vi "Subtask1_Marble_Project.vi"() -> ()   [LabVIEW 2016]
uses:
  <vilib>/NXT/Block Support/NXT_InputPort.ctl
  <vilib>/NXT/Block Support/NXT_OutputPort.ctl
  <vilib>/NXT/Dual Mode Library/Sensors/Touch_Pressed.vi
  <vilib>/NXT/Dual Mode Library/Sensors/Touch_Bumped.vi
  <vilib>/NXT/NXTIO Xnodes/NXTIONodeSubVIs/NXTMoveMotors.vi
  <vilib>/NXT/NXTIO Xnodes/AddressXNode/NXTIOAddress.xnode
  <vilib>/NXT/NXTIO Xnodes/NXTIOXNode/NXTIO.xnode
  <vilib>/NXT/Subs/LVHSConnector.ctl
  <vilib>/NXT/LegoClasses/BrickReference/BrickReference.lvclass
panel:
  out "Motor Power":dbl
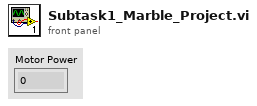
[diagram p1: front panel]
types:
  T1 = typedef "NXT_InputPort.ctl" = u32
  T2 = typedef "LVHSConnector.ctl" = refnum<class "BrickReference.lvclass">
  T3 = typedef "NXT_OutputPort.ctl" = u8
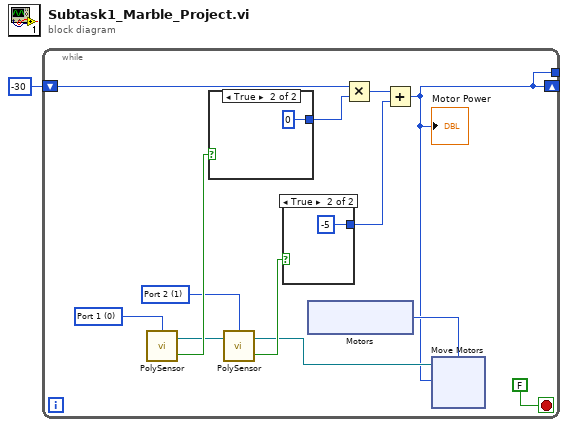
[diagram p0: block diagram]
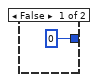
[diagram p2: hidden frame]
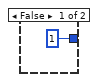
[diagram p3: hidden frame]
diagram:
  n1 = while {
    shift-right: [w2] -> _
    shift-left: -30 -> [w11]
    tunnel: [w2] -> _
    stop <- FALSE stop-if-true
    w6 = T1 1 items=["Port 1", "Port 2", "Port 3", "Port 4"] ("Port (Port 1)")
    w12 = T1 0 items=["Port 1", "Port 2", "Port 3", "Port 4"] ("Port (Port 1)")
    n2 = call-poly <vilib>:"PolySensor.vi"("Port (Port 1)"=w12) -> ("Yes / No"=w13:bool, "NXT/EV3"=w4:T2)  [unwired: 2 in]
    n3 = case shown="True" w13 {
      tunnel: [1 0] -> w10
      frame False {
      }
      frame True {
      }
    }
    n4 = call-poly <vilib>:"PolySensor.vi"("NXT/EV3"=w4, "Port (Port 1)"=w6) -> ("Yes / No"=w7:bool, "NXT/EV3"=w3:T2)  [unwired: 1 in]
    n5 = case shown="True" w7 {
      tunnel: [0 -5] -> w9
      frame False {
      }
      frame True {
      }
    }
    n6 = xnode "Motors"() -> ("Motor"=w14:T3)
    n7 = Multiply(x=w11, y=w10) -> (x*y=w8:i32)
    n8 = Add(x=w8, y=w9) -> (x+y=w2:i32)
    "Motor Power" <- w2
    n9 = xnode "Move Motors"("Power/Speed 1"=w2, "Motors"=w14, "NXT/EV3"=w3) -> ()  [unwired: 1 out]
  }
